vi "5.vi"() -> ()   [LabVIEW 2021]
panel:
  out "Numeric":u64
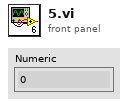
[diagram p1: front panel]
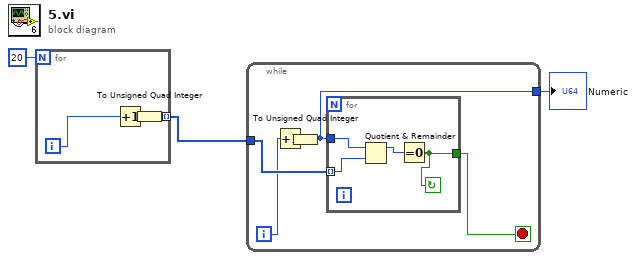
[diagram p0: block diagram]
diagram:
  n1 = for {
    N: 20 -> [_]
    tunnel: [w4] -> w2 mode=indexing
    i -> [w6]
    n2 = Increment(x=w6) -> (x+1=w5:i32)
    n3 = To Unsigned Quad Integer(1:w5) -> (0:w4:u64)
  }
  n4 = while {
    tunnel: w2 -> [w11]
    tunnel: [w7] -> w1
    i -> [w10]
    stop <- w8 stop-if-true
    n5 = Increment(x=w10) -> (x+1=w9:i32)
    n6 = To Unsigned Quad Integer(1:w9) -> (0:w7:u64)
    n7 = for {
      tunnel: w11 -> [w14] mode=indexing
      tunnel: w7 -> [w15]
      tunnel: [w12] -> w8
      stop <- w12 continue-if-true
      n8 = Quotient & Remainder(x=w15, y=w14) -> (x-y*floor(x/y)=w13:u64)  [unwired: 1 out]
      n9 = Equal To 0?(x=w13) -> (x = 0?=w12:bool)
    }
  }
  "Numeric" <- w1
